vi "选择功能.vi"(9 "错误输入（无错误）":errorcluster, 10 "功能":string, 11 "按钮":refnum<vi>) -> (0 "循环":bool, 1 "错误输出":errorcluster, 2 "正向":bool, 3 "功能输出":string, 6 "方向":string)   [LabVIEW 2020]
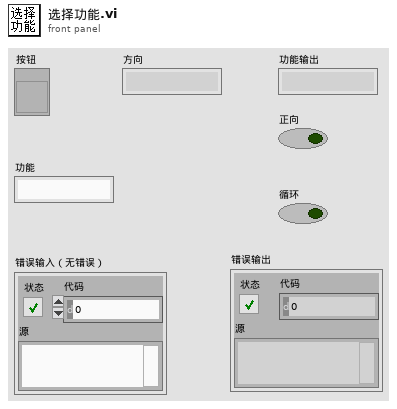
[diagram p1: front panel]
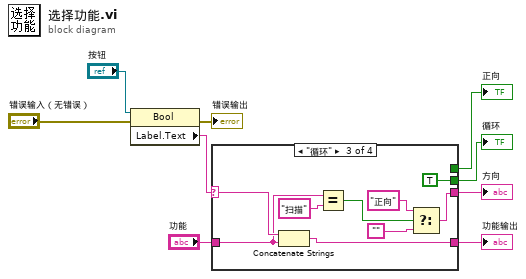
[diagram p0: block diagram]
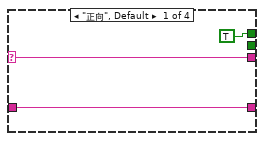
[diagram p2: hidden frame]
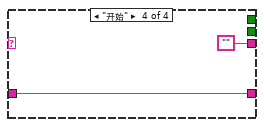
[diagram p4: hidden frame]
diagram:
  n1 = property class="Bool"(reference="按钮", error in="错误输入（无错误）") -> (error out=→"错误输出":errorcluster, "Label.Text"=w6:string)  [unwired: 1 out]
  n2 = case shown="\"循环\"" w6 {
    selector: w6 -> [w12 w14 w23 _]
    tunnel: [w12 w14 w19 ""] -> w5
    tunnel: [TRUE _ _ _] -> w4
    tunnel: [w10 w13 w22 w24] -> w3
    tunnel: "功能" -> [w10 w13 w17 w24]
    tunnel: [_ _ TRUE _] -> w1
    frame "正向", Default {
    }
    frame "负向" {
    }
    frame "循环" {
      n3 = Concatenate Strings(w23, w17) -> (w22:string)
      n4 = Equal?(x=w17, y="扫描") -> (x = y?=w15:bool)
      n5 = Select(t="正向" ("x"), s=w15, f="") -> (s? t:f=w19:string)
    }
    frame "开始" {
    }
  }
  "方向" <- w5
  "正向" <- w4
  "功能输出" <- w3
  "循环" <- w1
